vi "Emballage continue cmde en cours ss mélange.vi"(5 "n° cmde":string) -> (0 "Nb ds dernier carton":i32, 1 "n° dernier carton":u64, 2 "Tableau des lots déjà emballés":string[][](array[string]))   [LabVIEW 2020]
uses:
  Modules/FS/60_FS_Controles/60_FS_SetGet.ctl
panel:
  out "Tableau historique OUT":string[][](array[string])=[["112105740008090004", "01.01.2001 01:01:00", "55", "01234/08-01.01.01", "1", "0"], ["112105740008090006", "01.01.2001 01:01:00", "55", "56789/08-01.01.01", "3", "0"], ["112105740008090007", "01.01.2001 01:01:00", "55", "56789/08-01.01.01", "4", "0"], ["112105740008090007", "01.01.2001 01:01:00", "55", "00123/08-01.01.01", "2", "1"]]
  # "colonne 0 : n° des pièces (code bar 18 chiffres)\n     colonne 1 : date\n     colonne 2 : visa emballage (n°)\n     colonne 3 : n° commande (complet)\n     colonne 4 : n° carton\n     colonne 5 : n° retour"
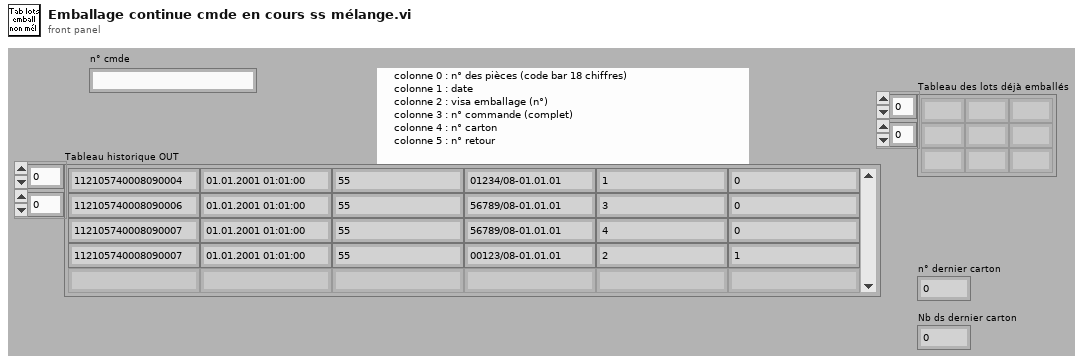
[diagram p1: front panel]
types:
  T1 = typedef "60_FS_SetGet.ctl" = enum16{"set", "get"}
  T2 = enum16{"n° produit", "date", "opérateur", "n° cmde", "n° carton"}
  T3 = typedef "Emballage_BDD_param_Produit.ctl" = cluster{"No_Valve_FAS":string, "suffixe":string, "designation":string, "indice_produit":string, "code_barre_fixe":string, "affiche_code_barre_client":string, "affiche_no_client":string, "Nb_vlve_par_carton":u16, "melange_des_lots_possible":string, "id_article":string, "Indice_Rev":string, "Famille":string, "date":string, "code_barre_fixe_Fin":string, "Longeur_No_Serie":string}
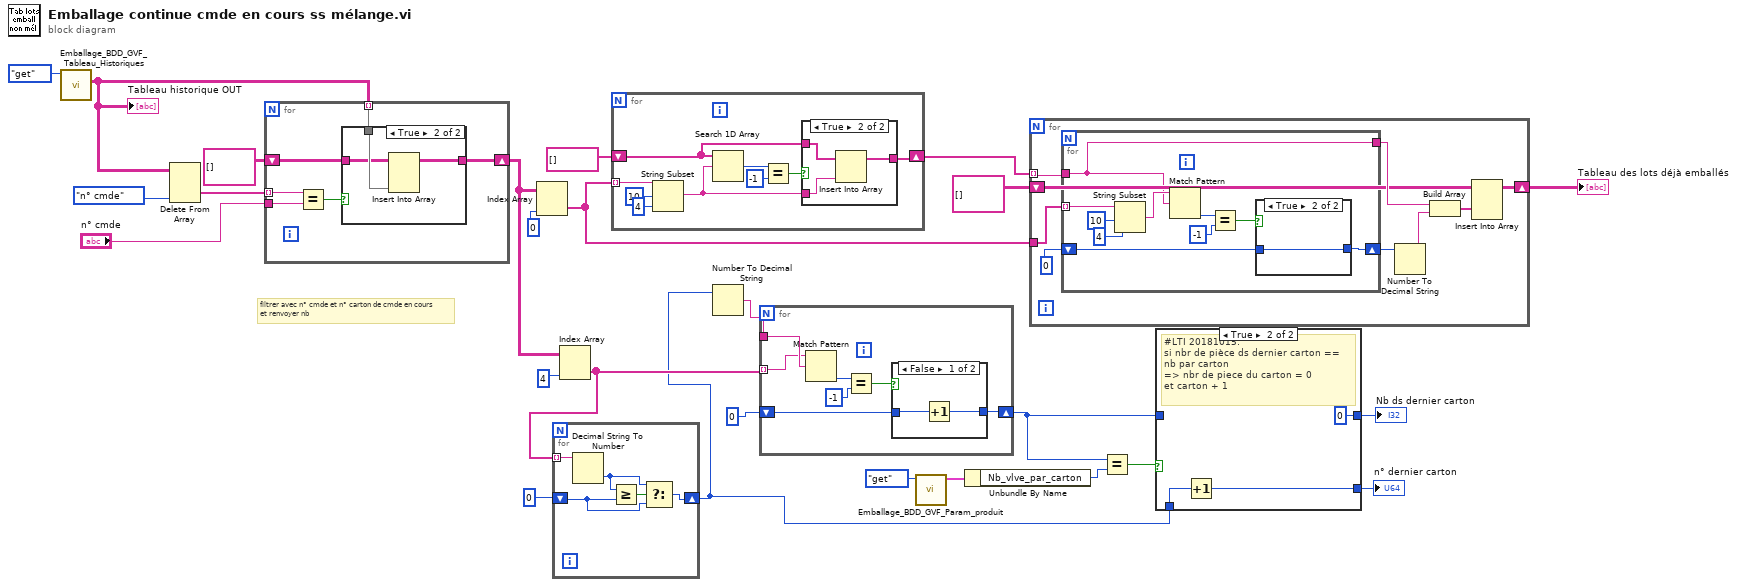
[diagram p0: block diagram]
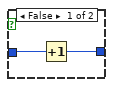
[diagram p4: hidden frame]
diagram:
  # "filtrer avec n° cmde et n° carton de cmde en cours\net renvoyer nb"
  n1 = call "Emballage_BDD_GVF_Tableau_Historiques.vi"("SetGet"=60_FS_SetGet."get") -> ("Tableau historique OUT"=w9:string[][])  [unwired: 9 in, 1 out]
  "Tableau historique OUT" <- w9
  n2 = Delete From Array(array=w9, index (col)=T2."n° cmde" ("Filtre")) -> (deleted portion=w26:string[])  [unwired: 2 in, 1 out]
  n3 = for {
    tunnel: w26 -> [w31] mode=indexing
    tunnel: "n° cmde" -> [w32]
    shift-right: [w28] -> w16
    shift-left: string[][] [] -> [w27]
    tunnel: w9 -> [w29] mode=indexing
    n4 = Equal?(x=w31, y=w32) -> (x = y?=w30:bool)
    n5 = case shown="True" w30 {
      tunnel: w29 -> [_ w36]
      tunnel: [w33 w35] -> w28
      tunnel: w27 -> [w33 w34]
      frame False {
      }
      frame True {
        n6 = Insert Into Array(array=w34, new element=w36) -> (w35:string[][])  [unwired: 2 in]
      }
    }
  }
  n7 = Index Array(array=w16, index (col)=0 ("indice désactivé (col)")) -> (element=w19:string[])  [unwired: 1 in]
  n8 = Index Array(array=w16, index (col)=4 ("indice désactivé (col)")) -> (element=w12:string[])  [unwired: 1 in]
  n9 = for {
    tunnel: w12 -> [w41] mode=indexing
    shift-right: [w37] -> w3
    shift-left: u64 0 -> [w38]
    n10 = Decimal String To Number(string=w41) -> (number=w39:i32)  [unwired: 2 in, 1 out]
    n11 = Greater Or Equal?(x=w39, y=w38) -> (x >= y?=w40:bool)
    n12 = Select(t=w39, s=w40, f=w38) -> (s? t:f=w37:u64)
  }
  n13 = for {
    tunnel: w19 -> [w45] mode=indexing
    shift-right: [w47] -> w20
    shift-left: string[] [] -> [w48]
    n14 = String Subset(string=w45, offset (0)=10, length (rest)=4 ("longueur (reste)")) -> (substring=w44:string)
    n15 = Search 1D Array(1D array=w48, element=w44) -> (index of element=w50:i32)  [unwired: 1 in]
    n16 = Equal?(x=w50, y=-1) -> (x = y?=w46:bool)
    n17 = case shown="True" w46 {
      tunnel: w44 -> [_ w53]
      tunnel: w48 -> [w51 w54]
      tunnel: [w51 w52] -> w47
      frame False {
      }
      frame True {
        n18 = Insert Into Array(array=w54, new element=w53) -> (w52:string[])  [unwired: 1 in]
      }
    }
  }
  n19 = Number To Decimal String(number=w3) -> (decimal integer string=w14:string)  [unwired: 1 in]
  n20 = for {
    tunnel: w12 -> [w55] mode=indexing
    tunnel: w14 -> [w56]
    shift-right: [w58] -> w5
    shift-left: u64 0 -> [w57]
    n21 = Match Pattern(string=w55, regular expression=w56) -> (offset past match=w61:i32)  [unwired: 1 in, 3 out]
    n22 = Equal?(x=w61, y=-1) -> (x = y?=w59:bool)
    n23 = case shown="False" w59 {
      tunnel: [w63 w64] -> w58
      tunnel: w57 -> [w62 w64]
      frame False {
        n24 = Increment(x=w62) -> (x+1=w63:u64)
      }
      frame True {
      }
    }
  }
  n25 = call "Emballage_BDD_GVF_Param_produit.vi"("Énum"=enum16{"set", "get"}."get") -> ("CLS_param_produit"=w8:T3)  [unwired: 7 in, 3 out]
  n26 = Unbundle By Name(w8) -> ("Nb_vlve_par_carton"=w2:u16)
  n27 = for {
    tunnel: w20 -> [w72] mode=indexing
    tunnel: w19 -> [w73]
    shift-right: [w66] -> w17
    shift-left: string[][] [] -> [w65]
    n28 = for {
      tunnel: w73 -> [w80] mode=indexing
      tunnel: w72 -> [w74]
      shift-right: [w76] -> w70
      shift-left: u64 0 -> [w75]
      tunnel: [w74] -> w68
      n29 = String Subset(string=w80, offset (0)=10, length (rest)=4 ("longueur (reste)")) -> (substring=w81:string)
      n30 = Match Pattern(string=w81, regular expression=w74) -> (offset past match=w79:i32)  [unwired: 1 in, 3 out]
      n31 = Equal?(x=w79, y=-1) -> (x = y?=w77:bool)
      n32 = case shown="True" w77 {
        tunnel: [w85 w86] -> w76
        tunnel: w75 -> [w84 w86]
        frame False {
          n33 = Increment(x=w84) -> (x+1=w85:u64)
        }
        frame True {
        }
      }
    }
    n34 = Number To Decimal String(number=w70) -> (decimal integer string=w69:string)  [unwired: 1 in]
    n35 = Build Array(w68, w69) -> (w67:string[])
    n36 = Insert Into Array(array=w65, new element=w67) -> (w66:string[][])  [unwired: 2 in]
  }
  "Tableau des lots déjà emballés" <- w17
  n37 = Equal?(x=w5, y=w2) -> (x = y?=w7:bool)
  n38 = case shown="True" w7 {
    tunnel: [w88 u64 0] -> w6
    tunnel: w5 -> [w88 _]
    tunnel: [w87 w89] -> w4
    tunnel: w3 -> [w87 w90]
    frame False {
    }
    frame True {
      # "#LTI 20181015:\nsi nbr de pièce ds dernier carton == nb par carton\n=> nbr de piece du carton = 0 \net carton + 1"
      n39 = Increment(x=w90) -> (x+1=w89:u64)
    }
  }
  "Nb ds dernier carton" <- w6
  "n° dernier carton" <- w4
